vi "Get All Folder VI Data--Class.vi"(8 "error in (no error)":errorcluster, 11 "Folder Path":path) -> (0 "error out":errorcluster, 3 "Item Data":refnum<class "Item.lvclass">[](array[class]))   [LabVIEW 2020, in "VI Properties Editor.lvlib"]
doc: "Gets all VI data from a folder located at <B>Path</B>."
uses:
  VI Properties Editor.lvlib
  Classes/Item/Item.lvclass
  Classes/Item Type.ctl
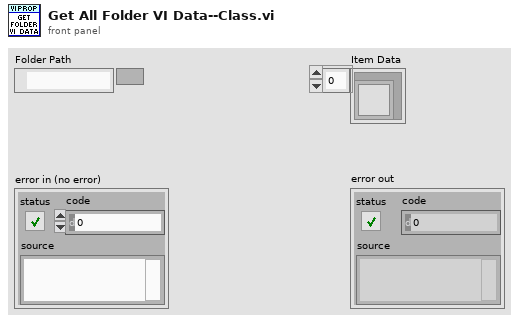
[diagram p1: front panel]
types:
  T1 = typedef "VI Properties Editor.lvlib/Item Type.ctl" = enum16{"VI"}
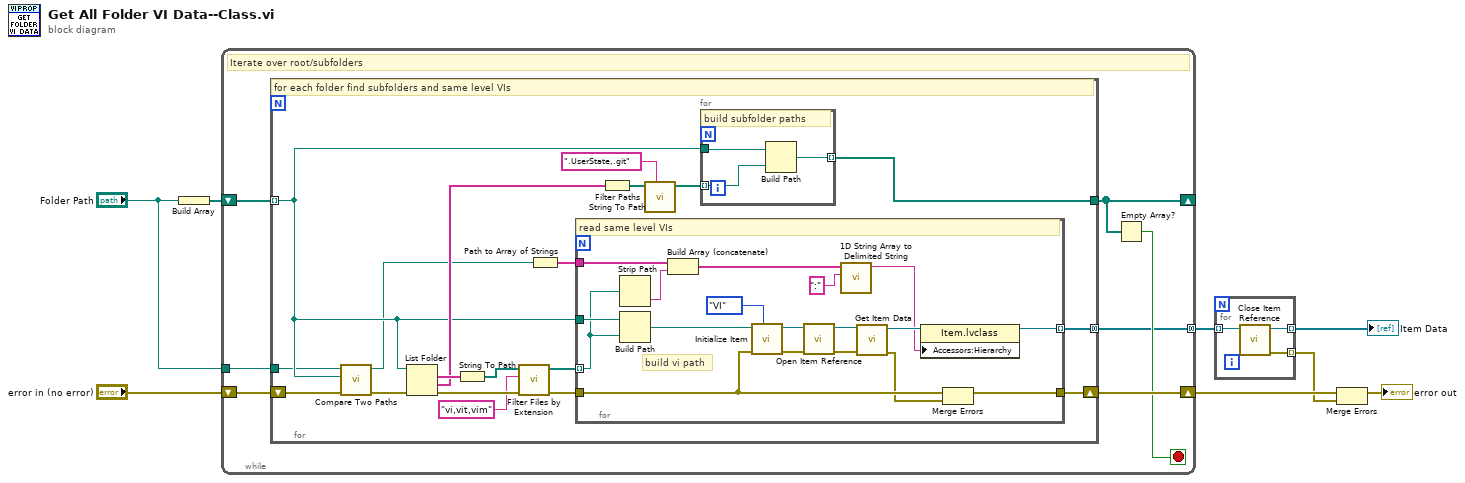
[diagram p0: block diagram]
diagram:
  n1 = Build Array("Folder Path") -> (w5:path[])
  n2 = while {
    shift-right: [w15] -> w7
    shift-left: "error in (no error)" -> [w14]
    shift-right: [w12] -> _
    shift-left: w5 -> [w13]
    tunnel: "Folder Path" -> [w10]
    tunnel: [w9] -> w3 mode=concatenating
    stop <- w11 stop-if-true
    # "Iterate over root/subfolders"
    n3 = for {
      tunnel: w13 -> [w20] mode=indexing
      shift-right: [w34] -> w15
      shift-left: w14 -> [w31]
      tunnel: [w27] -> w12
      tunnel: w10 -> [w19]
      tunnel: [w16] -> w9 mode=concatenating
      # "for each folder find subfolders and same level VIs"
      n4 = call <vilib>:"Compare Two Paths.vi"("error in (no error)"=w31, "Path 2"=w20, "Path 1"=w19) -> ("error out"=w30:errorcluster, "Relative Path from 1 to 2"=w18:path)  [unwired: 5 in, 2 out]
      n5 = List Folder(path=w20, error in=w30) -> (filenames=w29:string[], folder names=w24:string[], error out=w33:errorcluster)  [unwired: 2 in, 1 out]
      n6 = String To Path(string=w29) -> (path=w28:path[])
      n7 = call "Filter Files by Extension.vi"("error in (no error)"=w33, "Extensions"="vi,vit,vim", "Files"=w28) -> ("error out"=w32:errorcluster, "Files out"=w26:path[])  [unwired: 7 in]
      n8 = Path to Array of Strings(0:w18) -> (2:w17:string[])  [unwired: 1 out]
      n9 = for {
        tunnel: w32 -> [w51]
        tunnel: [w52] -> w34
        tunnel: w26 -> [w45] mode=indexing
        tunnel: w20 -> [w48]
        tunnel: w17 -> [w47]
        tunnel: [w38] -> w16 mode=indexing
        # "build vi path"
        # "read same level VIs"
        n10 = Strip Path(path=w45) -> (name=w43:string)  [unwired: 1 out]
        n11 = Build Path(base path=w48, name or relative path=w45) -> (appended path=w41:path)
        n12 = Build Array (concatenate)(w47, w43) -> (w44:string[])
        n13 = call "Initialize Item.vi"("Item Type"=Item_Type."VI", "error in (no error)"=w51, "Path"=w41) -> ("error out"=w50:errorcluster, "Item"=w36:refnum<class "Item.lvclass">)  [unwired: 7 in]
        n14 = call-dynamic "Open Item Reference.vi"("error in (no error)"=w50, "Item in"=w36) -> ("error out"=w37:errorcluster, "Item out"=w35:refnum<class "Item.lvclass">)  [unwired: 8 in]
        n15 = call <vilib>:"1D String Array to Delimited String.vi"("delimiter"=":", "string array"=w44) -> ("delimited string"=w39:string)  [unwired: 9 in]
        n16 = call-dynamic "Get Item Data.vi"("error in (no error)"=w37, "Item in"=w35) -> ("error out"=w49:errorcluster, "Item out"=w40:refnum<class "Item.lvclass">)  [unwired: 8 in]
        n17 = property class="Item.lvclass"(reference=w40, "Accessors:Hierarchy"=w39) -> (reference out=w38:refnum<class "Item.lvclass">)  [unwired: 1 in, 1 out]
        n18 = Merge Errors(w51, w49) -> (w52:errorcluster)
      }
      n19 = String To Path(string=w24) -> (path=w22:path[])
      n20 = call "Filter Paths.vi"("Argument"=".UserState,.git", "Paths"=w22) -> ("Filtered Path"=w23:path[])  [unwired: 9 in]
      n21 = for {
        tunnel: w20 -> [w54]
        tunnel: w23 -> [w55] mode=indexing
        tunnel: [w53] -> w27 mode=indexing
        # "build subfolder paths"
        n22 = Build Path(base path=w54, name or relative path=w55) -> (appended path=w53:path)
      }
    }
    n23 = Empty Array?(array=w12) -> (empty?=w11:bool)
  }
  n24 = for {
    tunnel: w3 -> [w57] mode=indexing
    tunnel: [w56] -> w2 mode=indexing
    tunnel: [w58] -> w1 mode=indexing
    n25 = call-dynamic "Close Item Reference.vi"("Item in"=w57) -> ("error out"=w58:errorcluster, "Item out"=w56:refnum<class "Item.lvclass">)  [unwired: 9 in]
  }
  "Item Data" <- w2
  n26 = Merge Errors(w7, w1) -> (→"error out":errorcluster)
